vi "Write Both Fan States.vi"(8 "error in (no error)":errorcluster, 9 "Fan B State":bool, 10 "Fan A State":bool, 11 "HW Dual Fan in":refnum<class "HW Dual Fan.lvclass">) -> (0 "error out":errorcluster)   [LabVIEW 2018, in "HW Dual Fan.lvclass"]
uses:
  HW Dual Fan.lvclass
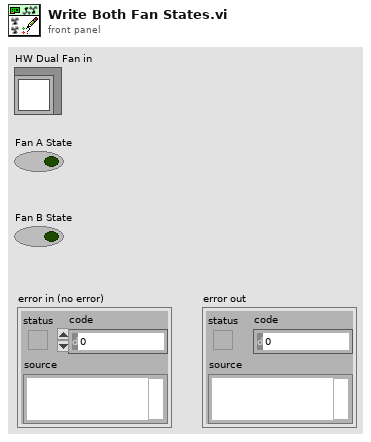
[diagram p1: front panel]
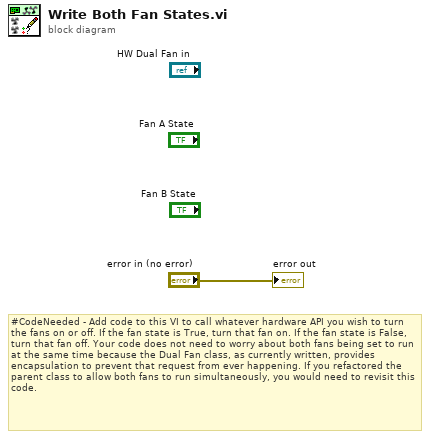
[diagram p0: block diagram]
diagram:
  # "#CodeNeeded - Add code to this VI to call whatever hardware API you wish to turn the fans on or off. If the fan state is True, turn that fan on. If the fan state is False, turn that fan off. Your code does not need to worry about both fans being set to run at the same time because the Dual Fan class, as currently written, provides encapsulation to prevent that request from ever happening. If you refactored the parent class to allow both fans to run simultaneously, you would need to revisit this code."
  "error out" <- "error in (no error)"
